vi "Memory.Pointer.Bool.Write.vi"(8 "error in (no error)":errorcluster, 10 "const value":bool, 11 "const Bool Pointer":refnum<class "Memory.Pointer.Bool.lvclass">) -> (0 "error out":errorcluster, 2 "value":bool, 3 "Bool Pointer":refnum<class "Memory.Pointer.Bool.lvclass">)   [LabVIEW 2016, in "Memory Manager.lvlib" / "Memory.Pointer.Bool.lvclass"]
uses:
  Memory.Pointer.Bool.lvclass
  C:/Users/Ryan/Documents/Git/Sourcetree/LabVIEW-Memory-Manager/Source/Library/Classes/Pointer/Pointer.Void/Memory.Pointer.Void.lvclass
  Pointer.Void/Memory.Pointer.Void.lvclass/Memory.Pointer.Void.ctl
  Pointer.Void/Memory.Pointer.Void.lvclass
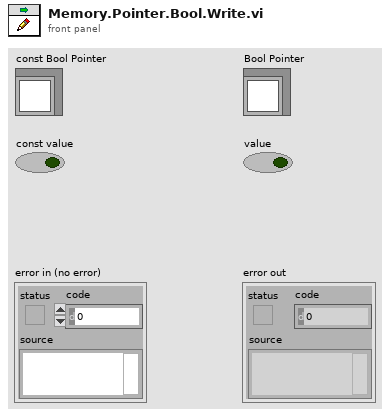
[diagram p1: front panel]
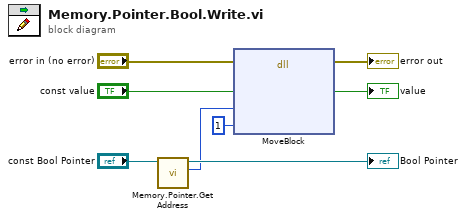
[diagram p0: block diagram]
diagram:
  n1 = call "Memory.Pointer.Get Address.vi"("Pointer in"="const Bool Pointer") -> ("address"=w1:u64, "Pointer out"=→"Bool Pointer":refnum<class "Memory.Pointer.Bool.lvclass">)  [unwired: 8 in, 1 out]
  n2 = dll-call lib="LabVIEW" fn="MoveBlock"(error in="error in (no error)", "src"="const value", "dst"=w1, "size"=u64 1) -> (error out=→"error out":errorcluster, "src"=→"value":bool)  [unwired: 5 in, 1 out]
